vi "test11.vi"() -> ()   [LabVIEW 2020]
panel:
  out "Array 4":dbl[](array[numeric])
  out "Array 3":dbl[](array[numeric])
  out "Array 2":i32[](array[numeric])
  out "Numeric":dbl
  in  "Array":dbl[](array[numeric])
  out "x/y":dbl
  out "appended array 2":dbl[](array[numeric])
  out "appended array 3":dbl[](array[numeric])
  in  "element 4":dbl
  in  "element":dbl
  out "appended array":dbl[](array[numeric])
  in  "element 3":dbl
  in  "element 1":dbl=2.0 format="%#_13g"
  in  "element 2":dbl
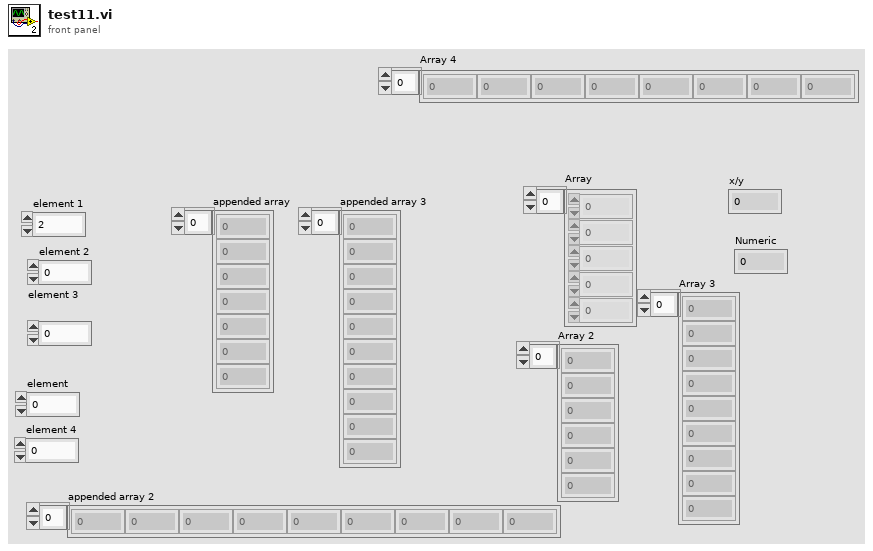
[diagram p1: front panel]
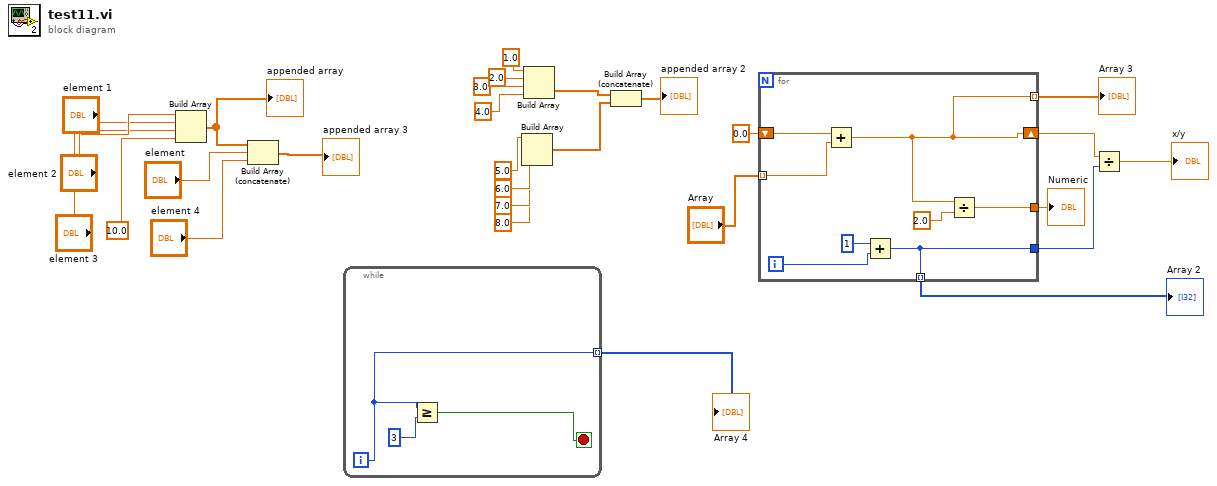
[diagram p0: block diagram]
diagram:
  n1 = Build Array("element 1", "element 2", "element 3", 10.0 ("element")) -> (w24:dbl[])
  "appended array" <- w24
  n2 = Build Array (concatenate)(w24, "element", "element 4") -> (→"appended array 3":dbl[])
  n3 = while {
    tunnel: [w31] -> w1 mode=indexing
    i -> [w31]
    stop <- w29 stop-if-true
    n4 = Greater Or Equal?(x=w31, y=3) -> (x >= y?=w29:bool)
  }
  "Array 4" <- w1
  n5 = Build Array(5.0 ("element"), 6.0 ("element"), 7.0 ("element"), 8.0 ("element")) -> (w11:dbl[])
  n6 = Build Array(1.0 ("element"), 2.0 ("element"), 3.0 ("element"), 4.0 ("element")) -> (w12:dbl[])
  n7 = Build Array (concatenate)(w12, w11) -> (→"appended array 2":dbl[])
  n8 = for {
    shift-right: [w32] -> w8
    shift-left: 0.0 -> [w39]
    tunnel: [w35] -> w4
    tunnel: [w33] -> w6
    tunnel: "Array" -> [w34] mode=indexing
    tunnel: [w33] -> w3 mode=indexing
    tunnel: [w32] -> w2 mode=indexing
    i -> [w37]
    n9 = Add(x=w39, y=w34) -> (x+y=w32:dbl)
    n10 = Add(x=1, y=w37) -> (x+y=w33:i32)
    n11 = Divide(x=w32, y=2.0) -> (x/y=w35:dbl)
  }
  "Numeric" <- w4
  "Array 2" <- w3
  "Array 3" <- w2
  n12 = Divide(x=w8, y=w6) -> (x/y=→"x/y":dbl)
